vi "Walk Down to Latest Build.vi"(8 "error in (no error)":errorcluster, 10 "name":string, 11 "Repository Path":path) -> (0 "error out":errorcluster, 3 "Latest Build Folder":path)   [LabVIEW 2019, in "Git.lvclass"]
uses:
  Git.lvclass
  <vilib>/Utility/error.llb/Error Cluster From Error Code.vi
  <vilib>/ErrorRing/Error Ring.xnode
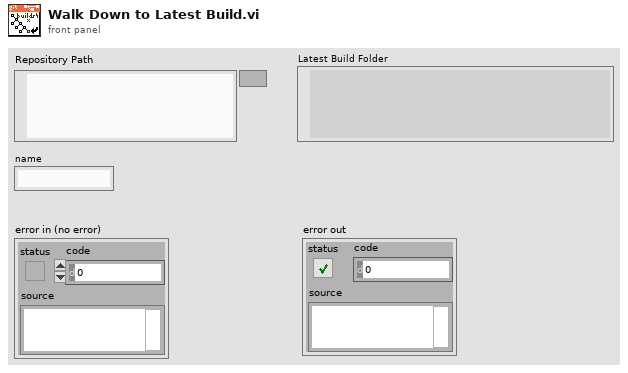
[diagram p1: front panel]
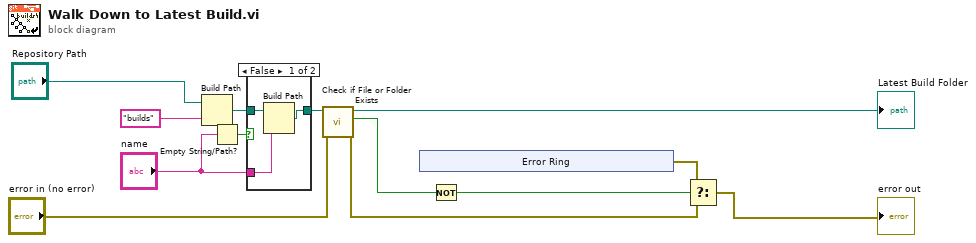
[diagram p0: block diagram]
diagram:
  n1 = Build Path(base path="Repository Path", name or relative path="builds") -> (appended path=w8:path)
  n2 = Empty String/Path?(string/path="name") -> (empty?=w5:bool)
  n3 = case shown="False" w5 {
    tunnel: w8 -> [w14 w17]
    tunnel: [w16 w17] -> w7
    tunnel: "name" -> [w15 _]
    frame False {
      n4 = Build Path(base path=w14, name or relative path=w15) -> (appended path=w16:path)
    }
    frame True {
    }
  }
  n5 = call <vilib>:"Check if File or Folder Exists.vi"("error in (no error)"="error in (no error)", "path"=w7) -> ("error out"=w4:errorcluster, "file or folder exists?"=w2:bool, "dup path"=→"Latest Build Folder":path)  [unwired: 7 in]
  n6 = xnode "Error Ring"() -> ("error out"=w3:errorcluster)
  n7 = Not(x=w2) -> (.not. x?=w1:bool)
  n8 = Select(t=w3, s=w1, f=w4) -> (s? t:f=→"error out":errorcluster)
